vi "thruster_dir_set.vi"(8 "Forward":bool, 9 "index":u16, 10 "Address":u16, 11 "VISA resource name":refnum<visa-resource-name>) -> ()   [LabVIEW 2014]
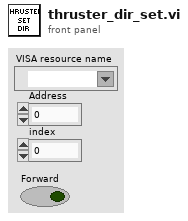
[diagram p1: front panel]
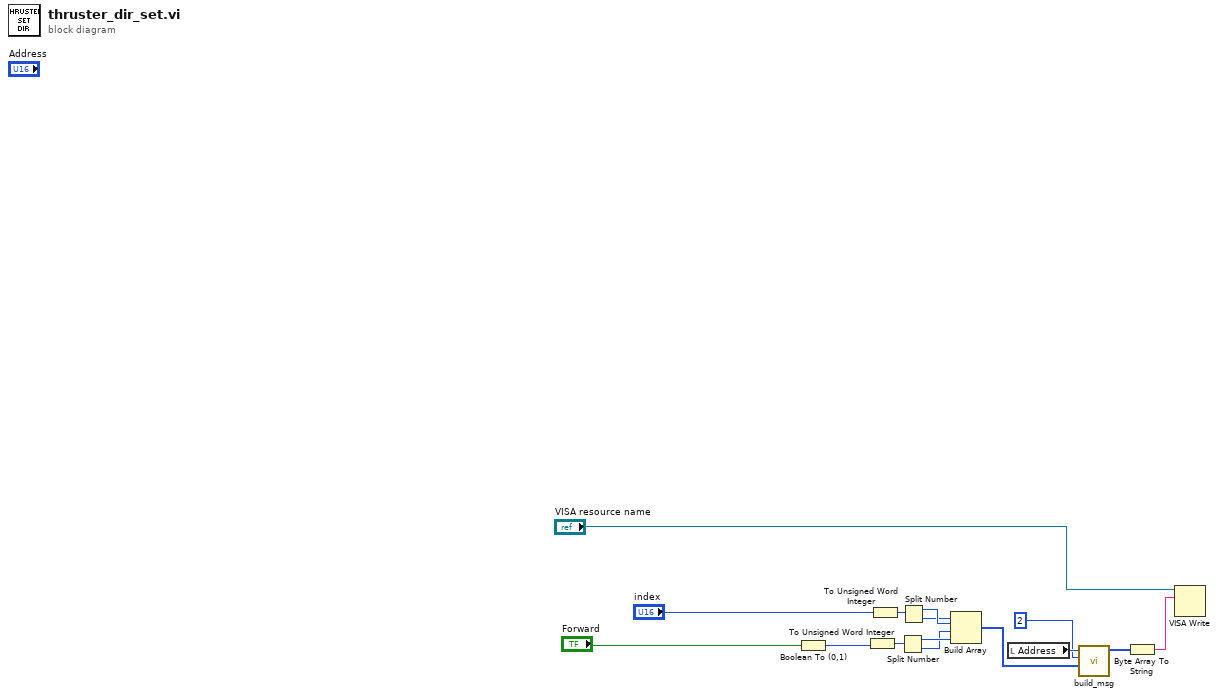
[diagram p0: block diagram]
diagram:
  n1 = Boolean To (0,1)(Boolean="Forward") -> (0, 1=w15:i16)
  n2 = To Unsigned Word Integer(number=w15) -> (unsigned 16bit integer=w7:u16)
  n3 = To Unsigned Word Integer(number="index") -> (unsigned 16bit integer=w13:u16)
  n4 = Split Number(x=w7) -> (hi(x)=w11:u8, lo(x)=w10:u8)
  n5 = Split Number(x=w13) -> (hi(x)=w9:u8, lo(x)=w8:u8)
  n6 = Build Array(w8, w9, w10, w11) -> (w12:u8[])
  n7 = local read "Address"() -> (w14:u16)
  n8 = call "build_msg.vi"("data"=w12, "ID"=u16 2, "Address"=w14) -> ("msg"=w5:u8[])  [unwired: 8 in]
  n9 = Byte Array To String(unsigned byte array=w5) -> (string=w4:string)
  n10 = VISA Write(VISA resource name="VISA resource name", write buffer=w4) -> ()  [unwired: 1 in, 3 out]
